vi "Sig-Override.vi"(8 "FJ":bool=TRUE, 9 "F0":bool=TRUE, 10 "F":bool=TRUE, 11 "BPCS-SIM-RX-ARRAY":dbl[](array[numeric])=[50.0, 50.0, 50.0]) -> ()   [LabVIEW 2018]
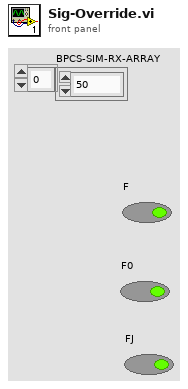
[diagram p1: front panel]
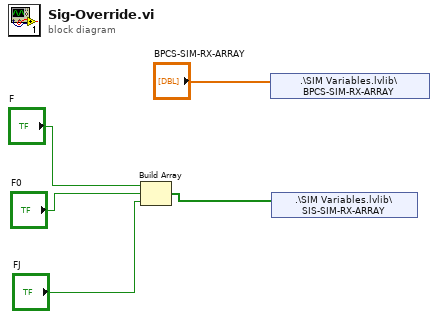
[diagram p0: block diagram]
diagram:
  n1 = Build Array("F", "F0", "FJ") -> (w1:bool[])
  n2 = shared-variable ".\\SIM Variables.lvlib\\BPCS-SIM-RX-ARRAY"("BPCS-SIM-RX-ARRAY") -> ()  [unwired: 1 in, 1 out]
  n3 = shared-variable ".\\SIM Variables.lvlib\\SIS-SIM-RX-ARRAY"(w1) -> ()  [unwired: 1 in, 1 out]
